vi "VG_TusineMin_P.vi"() -> ()   [LabVIEW 2020]
panel:
  out "TusineMin":dbl
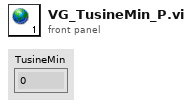
[diagram p1: front panel]
diagram:
